vi "LVData_measure.vi"(8 "error in (no error)":errorcluster, 10 "index":i32, 11 "LVData in":refnum<class "LVData.lvclass">) -> (0 "error out":errorcluster, 1 "Data acquired":dbl[](array[numeric]), 2 "Labels":string[](array[string]), 3 "LVData out":refnum<class "LVData.lvclass">)   [LabVIEW 2017, in "LVData.lvclass"]
uses:
  LVData.lvclass
  LVData.lvclass/LVData.ctl
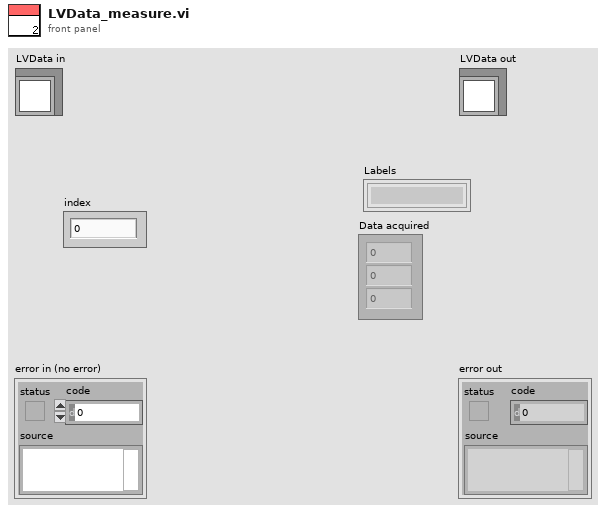
[diagram p1: front panel]
types:
  T1 = enum16{"Intialized", "Waiting", "Measuring", "Terminated"}
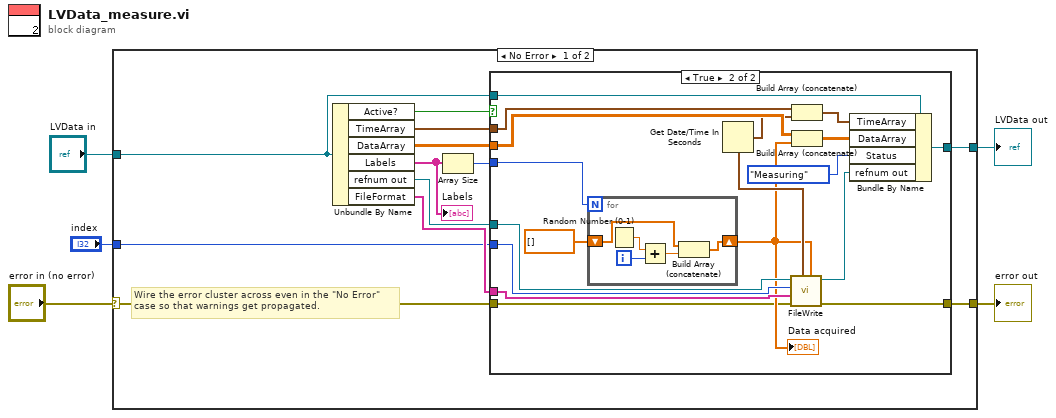
[diagram p0: block diagram]
diagram:
  n1 = case shown="No Error" "error in (no error)" {
    selector: "error in (no error)" -> [w7 w43]
    tunnel: [w6 w43] -> w4
    tunnel: [w15 w42] -> w2
    tunnel: "LVData in" -> [w17 w42]
    tunnel: "index" -> [w8 _]
    frame No Error {
      # "Wire the error cluster across even in the \"No Error\"\ncase so that warnings get propagated."
      n2 = Unbundle By Name(w17) -> ("Active?"=w16:bool, "TimeArray"=w14:timestamp[], "DataArray"=w13:dbl[][], "Labels"=w12:string[], "refnum out"=w10:refnum<file>, "FileFormat"=w9:string[])
      "Labels" <- w12
      n3 = Array Size(array=w12) -> (size(s)=w11:i32)
      n4 = case shown="True" w16 {
        tunnel: w17 -> [w19 w36]
        tunnel: [w19 w35] -> w15
        tunnel: w14 -> [_ w34]
        tunnel: w13 -> [_ w29]
        tunnel: w11 -> [_ w31]
        tunnel: w10 -> [_ w27]
        tunnel: w9 -> [_ w26]
        tunnel: w8 -> [_ w25]
        tunnel: w7 -> [w18 w22]
        tunnel: [w18 w21] -> w6
        frame False {
        }
        frame True {
          n5 = for {
            N: w31 -> [_]
            shift-right: [w38] -> w23
            shift-left: dbl[] [] -> [w39]
            i -> [w41]
            n6 = Random Number (0-1)() -> (number: 0 to 1=w40:dbl)
            n7 = Add(x=w40, y=w41) -> (x+y=w37:dbl)
            n8 = Build Array (concatenate)(w39, w37) -> (w38:dbl[])
          }
          "Data acquired" <- w23
          n9 = Get Date/Time In Seconds() -> (seconds since 1Jan1904=w24:timestamp)
          n10 = call "FileWrite.vi"("DataArray"=w23, "Time Stamp"=w24, "Error In"=w22, "FileFormat"=w26, "Index"=w25, "refnum in"=w27) -> ("Error Out"=w21:errorcluster, "Byte Stream File Refnum"=w20:refnum<file>)  [unwired: 4 in]
          n11 = Build Array (concatenate)(w34, w24) -> (w33:timestamp[])
          n12 = Build Array (concatenate)(w29, w23) -> (w28:dbl[][])
          n13 = Bundle By Name(cluster=w36, "TimeArray"=w33, "DataArray"=w28, "Status"=T1."Measuring", "refnum out"=w20) -> (w35:refnum<class "LVData.lvclass">)
        }
      }
    }
    frame Error {
    }
  }
  "error out" <- w4
  "LVData out" <- w2
